vi "NanotecSMCPD.get axis position.vi"(0 "i ref in":refnum<vi>, 1 "axis":i32, 3 "ms timeout (10000)":i32=10000, 5 "error in (no error)":errorcluster) -> (14 "i ref out":refnum<vi>, 15 "position [unit]":dbl=1.0, 17 "timed out":bool, 19 "error out":errorcluster)   [LabVIEW 2014, in "NanotecSMCPD.lvlib"]
doc: "Gets the value of the position counter of the specified axis."
uses:
  NanotecSMCPD.lvlib
  CS_Core/CSSystem/CoreDefs/CoreDefs.error_type.ctl
  CS_Core/CSSystem/CoreDefs/CoreDefs.error_severity.ctl
  CS_Core/CSApplicationBaseClasses/MotorBase/MotorBase.directionType.ctl
  CS_Core/CSApplicationBaseClasses/MotorBase/MotorBase.serviceType.ctl
  CSlibraries/UtilityLib/UtilityLib.valueStatus.ctl
  CS_Core/CSApplicationBaseClasses/DeviceBase/DeviceBase.lvlib
  CS_Core/CSSystem/CoreLib/CoreLib.lvlib
  CS_Core/CSApplicationBaseClasses/MotorBase/MotorBase.lvlib
  CSlibraries/UtilityLib/UtilityLib.lvlib
  instr.lib/NanotecSMCPD/NanotecSMCPDDriver.lvlib
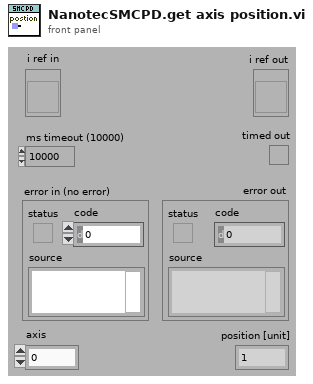
[diagram p1: front panel]
types:
  T1 = typedef "CoreDefs.error_severity.ctl" = enum16{"undefined", "information", "warning", "error", "fatal"}
  T2 = typedef "CoreDefs.error_type.ctl" = enum16{"no error", "can't load process", "can't unload process", "process does not exist", "can't install process", "can't remove process", "unknown function", "time out", "can't execute function", "duplicate queue name", "super not found", "caller queue invalid", "can't ping process", "unknown error", "VISA Error", "VISA timeout", "GPIB timeout", "GPIB error", "communication error", "data type mismatch", "can't read data from OPC server", "can't write data to OPC server", "OET error", "function not implemented", "process already exists", "invalid Shared Variable name", "error writing Shared Variable", "error reading Shared Variable", "invalid client name", "corrupt database", "unknown class", "call not authorized", "parameter out of range", "OET timeout: can't get data to modify", "invalid queue name", "requested operation incompatible with current state", "event undefined", "event disabled", "state undefined", "caller is not a friend", "EventBuilder: bad eventID", "EventBuilder: no DAQ devices", "a thread must not stop itself", "UNUSED ELEMENT4", "DiscArchiver: eventData incomplete", "DiscArchiver: eventData does not belong to run", "DiscArchiver: can't open file", "DiscArchiver: can't write to file", "DiscArchiver: available disc space low", "can't acquire semaphore", "error reading data from database", "notifier object is not existing", "can't register process", "can't unregister process", "illegal event type", "object disabled", "object already exists", "can't change state", "Instrument not found", "no connection to remote node", "invalid reference", "N/A", "UNUSED ELEMENT 1", "element not found", "illegal TCP/IP connection detected", "object does not exist", "invalid access ID", "unknown CS system", "invalid privilige", "unsupported data type", "unsupported server type", "IO server already exists", "Shared Variable already exists"}
  T3 = typedef "UtilityLib.lvlib/UtilityLib.valueStatus.ctl" = enum16{"no info available", "stand by/off", "on", "warning", "alarm/malfunction", "not implemented", "user action required", "important information", "system default", "control default", "indicator default", "button default"}
  T4 = typedef "MotorBase.lvlib/MotorBase.serviceType.ctl" = enum16{"onOff", "startVelocity", "stopVelocity", "acceleration", "rangeMin", "rangeMax", "status", "position"}
  T5 = typedef "MotorBase.lvlib/MotorBase.directionType.ctl" = enum16{"unknown", "update actual value", "update nominal value", "update both"}
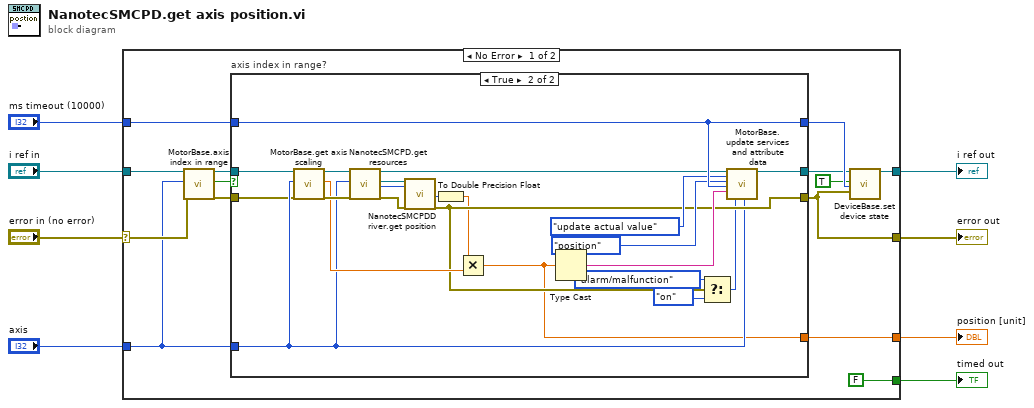
[diagram p0: block diagram]
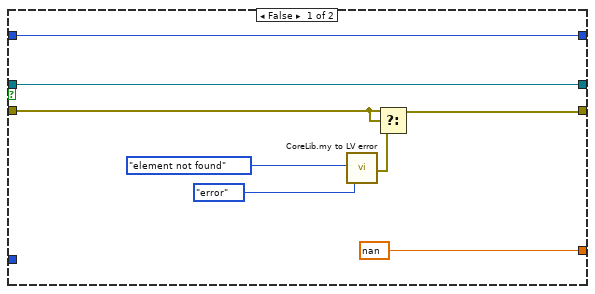
[diagram p2: hidden frame]
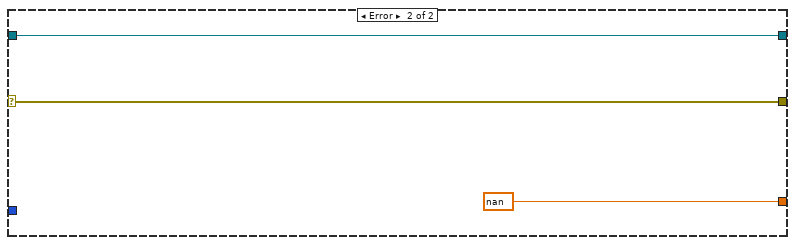
[diagram p3: hidden frame]
diagram:
  n1 = case shown="No Error" "error in (no error)" {
    selector: "error in (no error)" -> [w15 w54]
    tunnel: "ms timeout (10000)" -> [w12 _]
    tunnel: "i ref in" -> [w16 w55]
    tunnel: [w14 w54] -> w5
    tunnel: "axis" -> [w13 _]
    tunnel: [w11 w55] -> w3
    tunnel: [w10 nan] -> w2
    tunnel: [FALSE _] -> w1
    frame No Error {
      n2 = call "MotorBase.axis index in range.vi"("i ref in"=w16, "axisIndex"=w13, "error in (no error)"=w15) -> ("i ref out"=w20:refnum<vi>, "in range"=w19:bool, "error out"=w21:errorcluster)  [unwired: 14 in]
      n3 = case "axis index in range?" shown="True" w19 {
        tunnel: [w30 w38] -> w18
        tunnel: [w27 w40] -> w14
        tunnel: w12 -> [w24 w52]
        tunnel: w13 -> [_ w34]
        tunnel: w20 -> [w30 w31]
        tunnel: w21 -> [w28 w32]
        tunnel: [w24 w52] -> w22
        tunnel: [nan w33] -> w10
        frame False {
          n4 = call "CoreLib.my to LV error.vi"("ErrorTypes"=CoreDefs.error_type."element not found", "severityLevel"=CoreDefs.error_severity."error") -> ("myErrorCluster"=w26:errorcluster)  [unwired: 16 in, 1 out]
          n5 = Select(t=w28, s=w28, f=w26) -> (s? t:f=w27:errorcluster)
        }
        frame True {
          n6 = call "MotorBase.get axis scaling.vi"("i ref in"=w31, "axisIndex"=w34, "error in (no error)"=w32) -> ("i ref out"=w45:refnum<vi>, "scaling"=w43:dbl, "error out"=w44:errorcluster)  [unwired: 14 in]
          n7 = call "NanotecSMCPD.get resources.vi"("i ref in"=w45, "axisNumber"=w34, "error in (no error)"=w44) -> ("i ref out"=w46:refnum<vi>, "VISA resource"=w48:refnum<visa-resource-name>, "address"=w37:i32, "error out"=w47:errorcluster)  [unwired: 13 in]
          n8 = call "NanotecSMCPDDriver.get position.vi"("VISA resource name"=w48, "contollerID"=w37, "error in (no error)"=w47) -> ("actPosition [usteps]"=w36:i32, "error out"=w40:errorcluster)  [unwired: 13 in, 2 out]
          n9 = To Double Precision Float(number=w36) -> (double precision float=w35:dbl)
          n10 = Multiply(x=w35, y=w43) -> (x*y=w33:dbl)
          n11 = Type Cast(x=w33) -> (*(type *) &x=w51:string)  [unwired: 1 in]
          n12 = Select(t=UtilityLib.valueStatus."alarm/malfunction", s=w40, f=UtilityLib.valueStatus."on" ("quality")) -> (s? t:f=w39:T3)
          n13 = call "MotorBase.update services and attribute data.vi"("i ref in"=w46, "direction"=MotorBase.directionType."update actual value", "service"=MotorBase.serviceType."position", "ms timeout (10000)"=w52, "value"=w51, "quality"=w39, "axisNumber"=w34) -> ("i ref out"=w38:refnum<vi>)  [unwired: 10 in, 2 out]
        }
      }
      n14 = call "DeviceBase.set device state.vi"("i ref in"=w18, "implicit"=TRUE, "ms timeout (10000)"=w22, "device error"=w14) -> ("i ref out"=w11:refnum<vi>)  [unwired: 13 in, 2 out]
    }
    frame Error {
    }
  }
  "error out" <- w5
  "i ref out" <- w3
  "timed out" <- w1
  "position [unit]" <- w2
